vi "lr1v1.vi"() -> ()   [LabVIEW 2012]
uses:
  <vilib>/express/express arith-compare/Formula/XNode/ExpressFormulaBlockNode.xnode
panel:
  out "Thermometer 2":dbl(slide) scale=-50.0..50.0
  in  "Boolean":bool
  out "Thermometer":dbl(slide) scale=-50.0..50.0
  in  "Slide":dbl(slide) scale=-60.0..130.0
  # "F"
  # "C"
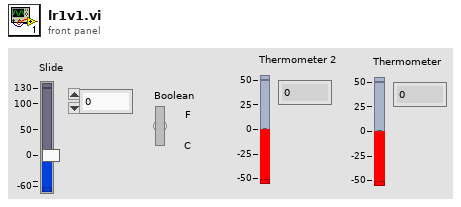
[diagram p1: front panel]
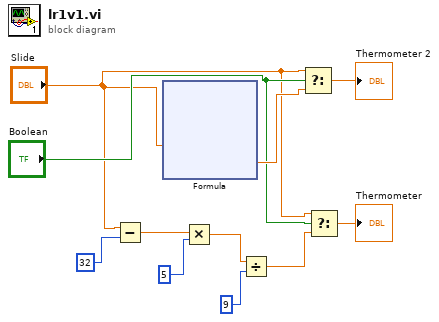
[diagram p0: block diagram]
diagram:
  n1 = Subtract(x="Slide", y=32) -> (x-y=w5:dbl)
  n2 = xnode "Formula"("T"="Slide") -> ("Result"=w9:dbl)  [unwired: 1 in, 1 out]
  n3 = Multiply(x=w5, y=5) -> (x*y=w3:dbl)
  n4 = Divide(x=w3, y=9) -> (x/y=w1:dbl)
  n5 = Select(t="Slide", s="Boolean", f=w9) -> (s? t:f=→"Thermometer 2":dbl)
  n6 = Select(t="Slide", s="Boolean", f=w1) -> (s? t:f=→"Thermometer":dbl)
